vi "Stack1LUT(SubVI).vi"(2 "Array":dbl[][][](array[numeric]), 3 "LUT image data path 2":path) -> (0 "Stacked LUTs":dbl[][][](array[numeric]), 1 "Intensity Graph":dbl[][](graph))   [LabVIEW 2011]
uses:
  <vilib>/Utility/file.llb/Read From Spreadsheet File (DBL).vi
panel:
  out "size(s)":i32[](array[numeric])
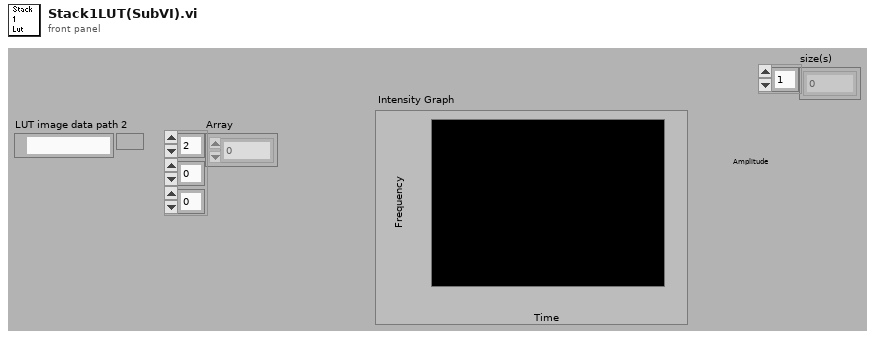
[diagram p1: front panel]
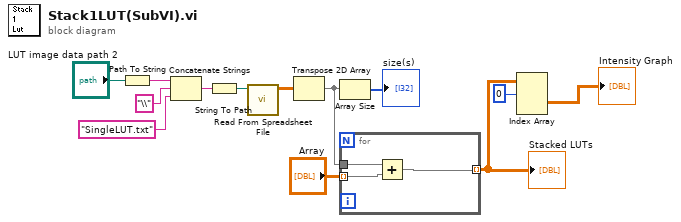
[diagram p0: block diagram]
diagram:
  n1 = Path To String(path="LUT image data path 2") -> (string=w12:string)
  n2 = Concatenate Strings(w12, "\\", "SingleLUT.txt") -> (w9:string)
  n3 = String To Path(string=w9) -> (path=w8:path)
  n4 = call-poly <vilib>:"Read From Spreadsheet File.vi"("file path (dialog if empty)"=w8) -> ("all rows"=w2:dbl[][])  [unwired: 3 in, 7 out]
  n5 = Transpose 2D Array(2D array=w2) -> (transposed array=w1:dbl[][])
  n6 = Array Size(array=w1) -> (size(s)=→"size(s)":i32[])
  n7 = for {
    tunnel: "Array" -> [w15] mode=indexing
    tunnel: w1 -> [w16]
    tunnel: [w14] -> w7 mode=indexing
    n8 = Add(x=w16, y=w15) -> (x+y=w14:dbl[][])
  }
  "Stacked LUTs" <- w7
  n9 = Index Array(array=w7, index (dim 0)=0 ("index (page)")) -> (element=→"Intensity Graph":dbl[][])  [unwired: 2 in]
